vi "getAllsubset.vi"(8 "error in (no error)":errorcluster, 10 "getAll":T1, 11 "instrument.PPMS2 in":refnum<class "instrument.PPMS2.lvclass">) -> (0 "error out":errorcluster, 2 "output cluster":variant, 3 "instrument.PPMS2 out":refnum<class "instrument.PPMS2.lvclass">)   [LabVIEW 2019, in "instrument.PPMS2.lvclass"]
uses:
  instrument.PPMS2.lvclass
  instrument.PPMS/Typedefs/PPMS.getAll--cluster.ctl
  instrument.PPMS/instrument.PPMS.lvclass
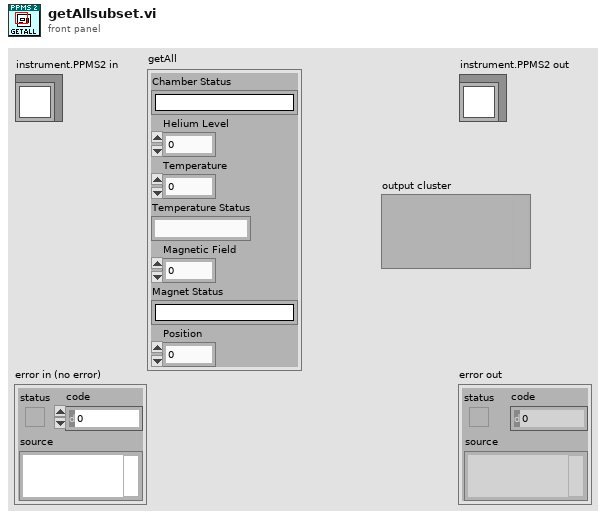
[diagram p1: front panel]
types:
  T1 = typedef "instrument.PPMS.lvclass/PPMS.getAll--cluster.ctl" = cluster{"Chamber Status":string, "Helium Level":dbl, "Temperature":dbl, "Temperature Status":string, "Magnetic Field":dbl, "Magnet Status":string, "Position":dbl}
  T2 = cluster{"Chamber Status":string, "Helium Level":dbl, "Temperature":dbl, "Temperature Status":string, "Magnetic Field":dbl, "Magnet Status":string, "Position":dbl}
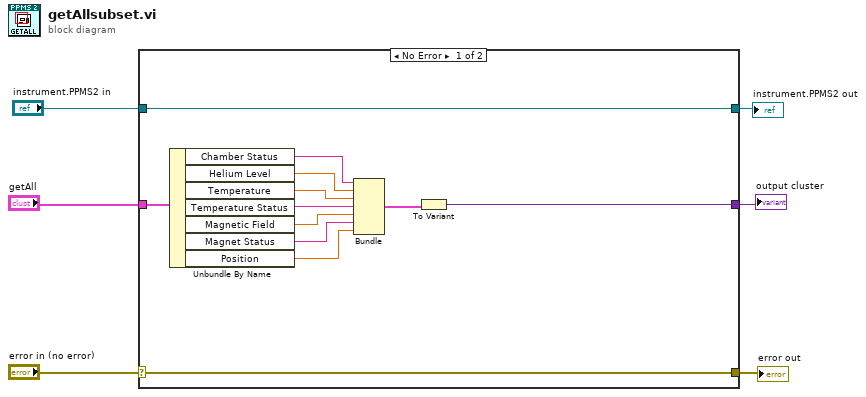
[diagram p0: block diagram]
diagram:
  n1 = case shown="No Error" "error in (no error)" {
    selector: "error in (no error)" -> [w17 w20]
    tunnel: [w17 w20] -> w4
    tunnel: [w18 w19] -> w6
    tunnel: "instrument.PPMS2 in" -> [w18 w19]
    tunnel: "getAll" -> [w8 _]
    tunnel: [w16 _] -> w5
    frame No Error {
      n2 = Unbundle By Name(w8) -> ("Chamber Status"=w10:string, "Helium Level"=w13:dbl, "Temperature"=w14:dbl, "Temperature Status"=w15:string, "Magnetic Field"=w12:dbl, "Magnet Status"=w11:string, "Position"=w9:dbl)
      n3 = Bundle("Chamber Status"=w10, "Helium Level"=w13, "Temperature"=w14, "Temperature Status"=w15, "Magnetic Field"=w12, "Magnet Status"=w11, "Position"=w9) -> (w7:T2)  [unwired: 1 in]
      n4 = To Variant(anything=w7) -> (Variant=w16:variant)
    }
    frame Error {
    }
  }
  "error out" <- w4
  "instrument.PPMS2 out" <- w6
  "output cluster" <- w5
